vi "Cal6-MakeLabels.vi"() -> (1 "String":string, 2 "String 2":string, 3 "Boolean":bool, 4 "Array":string[](array[string]), 5 "Boolean 2":bool, 6 "Boolean 3":bool)   [LabVIEW 2020]
uses:
  Anemometry Sub Vis/Globals/Calib_global.vi
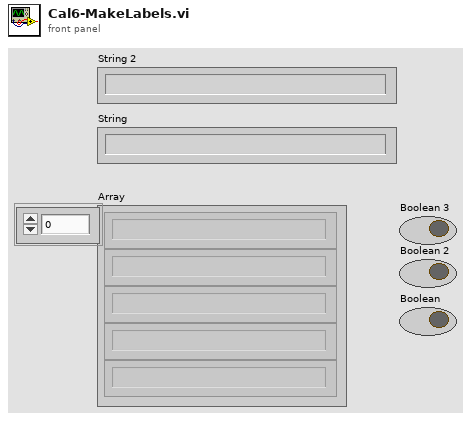
[diagram p1: front panel]
types:
  T1 = typedef "Ref_Inst_type.ctl" = enum16{"Propellor anemometer", "Pressure Transducer", "Raw voltage", "Pitot-static tube", "Generic Linear", "Generic Polynomial", "Thermocouple", "LDA", "Enter Value", "ADAM Channel"}
  T2 = typedef "Cal_Inst_type.ctl" = enum16{"Propeller anemometer", "Pressure Transducer", "Hot wire", "Cross wire velocity", "Cross wire angle", "Generic Linear", "Generic Polynomial", "Generic BackPoly", "Fast FID", "Thermocouple", "Cold wire", "Pulsed Wire"}
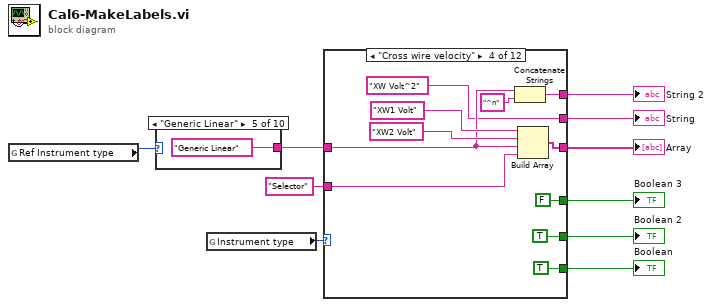
[diagram p0: block diagram]
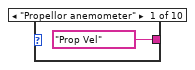
[diagram p2: hidden frame]
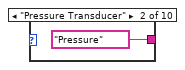
[diagram p3: hidden frame]
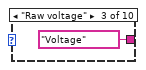
[diagram p4: hidden frame]
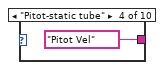
[diagram p5: hidden frame]
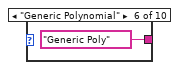
[diagram p6: hidden frame]
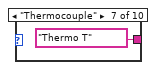
[diagram p7: hidden frame]
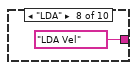
[diagram p8: hidden frame]
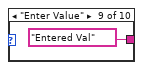
[diagram p9: hidden frame]
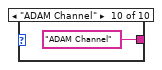
[diagram p10: hidden frame]
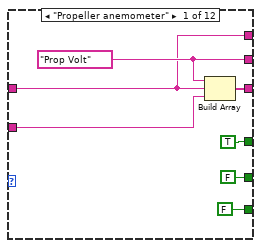
[diagram p11: hidden frame]
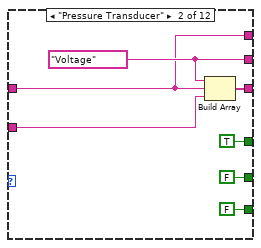
[diagram p12: hidden frame]
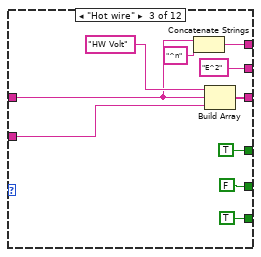
[diagram p13: hidden frame]
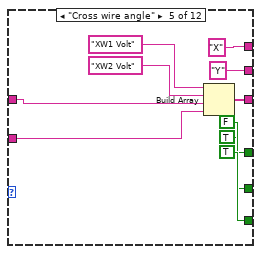
[diagram p14: hidden frame]
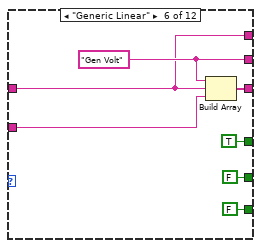
[diagram p15: hidden frame]
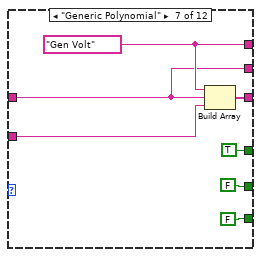
[diagram p16: hidden frame]
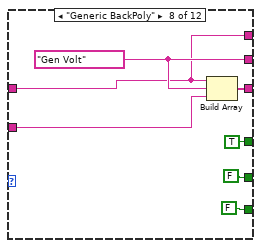
[diagram p17: hidden frame]
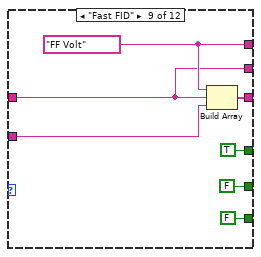
[diagram p18: hidden frame]
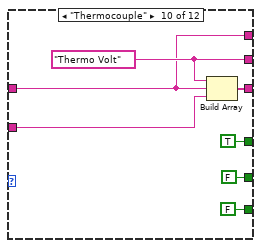
[diagram p19: hidden frame]
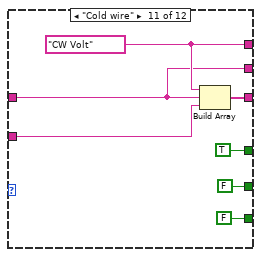
[diagram p20: hidden frame]
diagram:
  n1 = global read "Calib_global.vi" "Ref Instrument type"() -> (w7:T1)
  n2 = case shown="\"Generic Linear\"" w7 {
    tunnel: ["Prop Vel" "Pressure" "Voltage" "Pitot Vel" "Generic Linear" "Generic Poly" "Thermo T" "LDA Vel" "Entered Val" "ADAM Channel"] -> w4
    frame "Propellor anemometer" {
    }
    frame "Pressure Transducer" {
    }
    frame "Raw voltage" {
    }
    frame "Pitot-static tube" {
    }
    frame "Generic Linear" {
    }
    frame "Generic Polynomial" {
    }
    frame "Thermocouple" {
    }
    frame "LDA" {
    }
    frame "Enter Value" {
    }
    frame "ADAM Channel" {
    }
  }
  n3 = global read "Calib_global.vi" "Instrument type"() -> (w6:T2)
  n4 = case shown="\"Cross wire velocity\"" w6 {
    tunnel: [FALSE FALSE TRUE TRUE TRUE FALSE FALSE FALSE FALSE FALSE FALSE FALSE] -> w10
    tunnel: [TRUE TRUE TRUE FALSE FALSE TRUE TRUE TRUE TRUE TRUE TRUE TRUE] -> w2
    tunnel: [FALSE FALSE FALSE TRUE TRUE FALSE FALSE FALSE FALSE FALSE FALSE FALSE] -> w3
    tunnel: w4 -> [w21 w28 w37 w47 w57 w67 w73 w80 w87 w95 w101 w108]
    tunnel: [w24 w31 w40 w50 w60 w69 w76 w83 w90 w97 w104 w111] -> w5
    tunnel: "Selector" -> [w23 w30 w39 w49 w59 w66 w75 w82 w89 w94 w103 w110]
    tunnel: [w22 w29 "E^2" "XW Volt^2" "Y" w68 w73 w81 w87 w96 w101 w108] -> w9
    tunnel: [w21 w28 w35 w45 "X" w67 w74 w80 w88 w95 w102 w109] -> w8
    frame "Propeller anemometer" {
      w22 = "Prop Volt"
      n5 = Build Array(w22, w21, w23) -> (w24:string[])
    }
    frame "Pressure Transducer" {
      w29 = "Voltage"
      n6 = Build Array(w29, w28, w30) -> (w31:string[])
    }
    frame "Hot wire" {
      n7 = Concatenate Strings(w37, "^n") -> (w35:string)
      n8 = Build Array("HW Volt", w37, w39) -> (w40:string[])
    }
    frame "Cross wire velocity" {
      n9 = Concatenate Strings(w47, "^n") -> (w45:string)
      n10 = Build Array("XW1 Volt", "XW2 Volt", w47, w49) -> (w50:string[])
    }
    frame "Cross wire angle" {
      n11 = Build Array("XW1 Volt", "XW2 Volt", w57, w59) -> (w60:string[])
    }
    frame "Generic Linear" {
      w68 = "Gen Volt"
      n12 = Build Array(w68, w67, w66) -> (w69:string[])
    }
    frame "Generic Polynomial" {
      w74 = "Gen Volt"
      n13 = Build Array(w74, w73, w75) -> (w76:string[])
    }
    frame "Generic BackPoly" {
      w81 = "Gen Volt"
      n14 = Build Array(w80, w81, w82) -> (w83:string[])
    }
    frame "Fast FID" {
      w88 = "FF Volt"
      n15 = Build Array(w88, w87, w89) -> (w90:string[])
    }
    frame "Thermocouple" {
      w96 = "Thermo Volt"
      n16 = Build Array(w96, w95, w94) -> (w97:string[])
    }
    frame "Cold wire" {
      w102 = "CW Volt"
      n17 = Build Array(w102, w101, w103) -> (w104:string[])
    }
    frame "Pulsed Wire" {
      w109 = "1/TOF"
      n18 = Build Array(w109, w108, w110) -> (w111:string[])
    }
  }
  "Boolean" <- w10
  "String" <- w9
  "String 2" <- w8
  "Array" <- w5
  "Boolean 2" <- w3
  "Boolean 3" <- w2
